vi "MenuDo.vi"(0 "GroupCol in":refnum<class "GroupCol.lvclass">, 1 "Column Array":refnum<vi>, 2 "Layout Ring Refnum":refnum<vi>, 3 "Clipboard":refnum<vi>, 5 "ItemTag":string, 7 "VariableManagerRef":refnum<vi>, 9 "Table CtlRef In":refnum<vi>, 11 "error in (no error)":errorcluster, 12 "Cell Position":T1, 13 "ModeCol Index":i32=2, 14 "Table History ref":refnum<vi>) -> (4 "GroupCol out":refnum<class "GroupCol.lvclass">, 6 "Col Array Ref out":refnum<vi>, 8 "Update HWI?":bool, 10 "Table CtlRef Out":refnum<vi>, 15 "error out":errorcluster)   [LabVIEW 2013, in "GroupCol.lvclass"]
doc: "Perform selected shortcut (right-click) menu actions for Group column.\nThis VI is read-only w.r.t column data."
uses:
  GroupCol.lvclass
  <vilib>/Utility/miscctls.llb/LVRowAndColumnTypeDef.ctl
  TypeDefs/TableHistory.ctl
  TypeDefs/TableArray.ctl
  VariableManagerCodes/VariableManager/VariableManager.lvclass
  DigitalCol/DigitalCol.lvclass
  Globals/StdRowHeightGlobal.vi
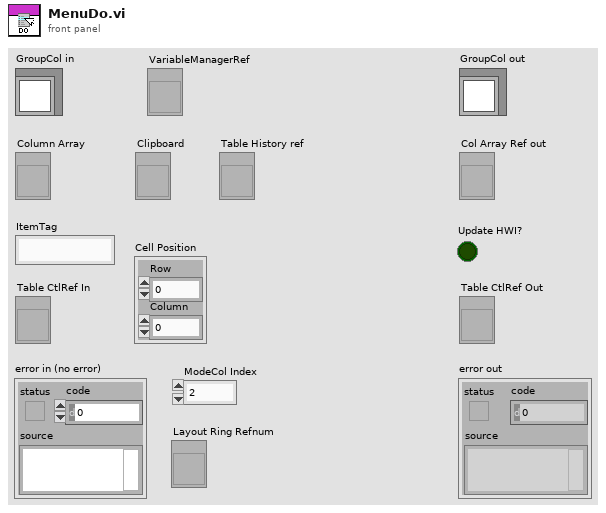
[diagram p1: front panel]
types:
  T1 = typedef "LVRowAndColumnTypeDef.ctl" = cluster{"Row":i32, "Column":i32}
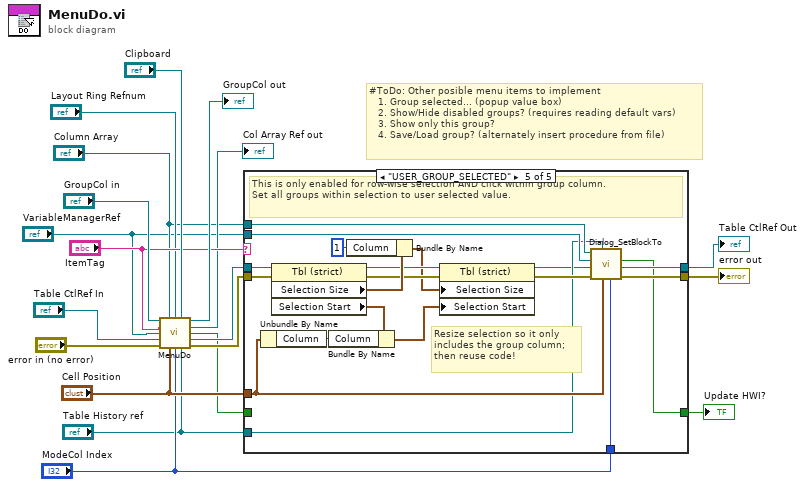
[diagram p0: block diagram]
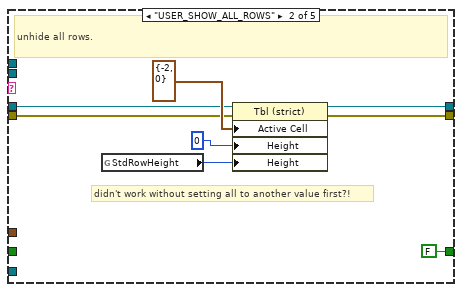
[diagram p3: hidden frame]
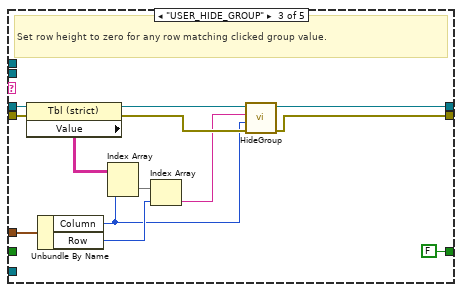
[diagram p4: hidden frame]
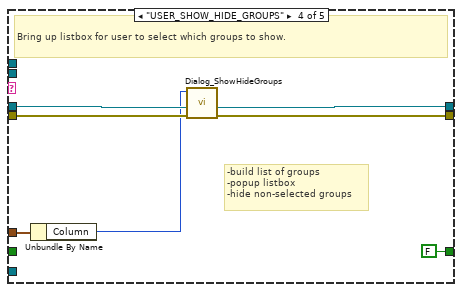
[diagram p5: hidden frame]
diagram:
  # "#ToDo: Other posible menu items to implement\n   1. Group selected... (popup value box)\n   2. Show/Hide disabled groups? (requires reading default vars)\n   3. Show only this group?\n   4. Save/Load group? (alternately insert procedure from file)"
  n1 = call-parent "MenuDo.vi"("DigitalCol in"="GroupCol in", "Column Array"="Column Array", "Layout Ring Refnum"="Layout Ring Refnum", "Clipboard"="Clipboard", "ItemTag"="ItemTag", "VariableManagerRef"="VariableManagerRef", "Table CtlRef In"="Table CtlRef In", "error in (no error)"="error in (no error)", "Cell Position"="Cell Position", "ModeCol Index"="ModeCol Index", "Table History ref"="Table History ref") -> ("DigitalCol out"=→"GroupCol out":refnum<class "GroupCol.lvclass">, "Col Array Ref out"=→"Col Array Ref out":refnum<vi>, "Update HWI?"=w2:bool, "Table CtlRef Out"=w9:refnum<vi>, "error out"=w10:errorcluster)
  n2 = case shown="\"USER_GROUP_SELECTED\"" "ItemTag" {
    tunnel: w9 -> [w22 w27 w42 w50 w69]
    tunnel: w10 -> [w21 w26 w39 w49 w68]
    tunnel: [w21 w30 w32 w48 w58] -> w19
    tunnel: [w22 w29 w43 w47 w52] -> w18
    tunnel: "Cell Position" -> [_ _ w36 w46 w57]
    tunnel: "ModeCol Index" -> [_ _ _ _ w56]
    tunnel: "Column Array" -> [_ _ _ _ w55]
    tunnel: "VariableManagerRef" -> [_ _ _ _ w54]
    tunnel: "Table History ref" -> [_ _ _ _ w53]
    tunnel: w2 -> [w20 _ _ _ _]
    tunnel: [w20 FALSE ("Update HWI?") FALSE ("Update HWI?") FALSE ("Update HWI?") w51] -> w1
    frame Default {
    }
    frame "USER_SHOW_ALL_ROWS" {
      # "didn't work without setting all to another value first?!"
      # "unhide all rows."
      n3 = global read "StdRowHeightGlobal.vi" "StdRowHeight"() -> (w25:u32)
      n4 = property class="Tbl (strict)"(reference=w27, error in=w26, "Active Cell"=T1 {"Row"=-2, "Column"=0} ("Active Cell:Active Cell"), "Height"=u32 0 ("Active Cell:Cell Size:Height"), "Height"=w25) -> (reference out=w29:refnum<vi>, error out=w30:errorcluster)
    }
    frame "USER_HIDE_GROUP" {
      # "Set row height to zero for any row matching clicked group value."
      n5 = property class="Tbl (strict)"(reference=w42, error in=w39) -> (reference out=w41:refnum<vi>, error out=w40:errorcluster, "Value"=w38:string[][])
      n6 = Unbundle By Name(w36) -> ("Column"=w33:i32, "Row"=w35:i32)
      n7 = Index Array(array=w38, index (col)=w33) -> (element=w37:string[])  [unwired: 1 in]
      n8 = Index Array(array=w37, index=w35) -> (element=w34:string)
      n9 = call "HideGroup.vi"("error in (no error)"=w40, "GroupCol Index"=w33, "String toHide"=w34, "Table CtlRef In"=w41) -> ("error out"=w32:errorcluster, "Table CtlRef Out"=w43:refnum<vi>)  [unwired: 6 in]
    }
    frame "USER_SHOW_HIDE_GROUPS" {
      # "-build list of groups\n-popup listbox\n-hide non-selected groups"
      # "Bring up listbox for user to select which groups to show."
      n10 = Unbundle By Name(w46) -> ("Column"=w45:i32)
      n11 = call "Dialog_ShowHideGroups.vi"("error in (no error)"=w49, "Table CtlRef In"=w50, "GroupCol Index"=w45) -> ("error out"=w48:errorcluster, "Table CtlRef Out"=w47:refnum<vi>)  [unwired: 7 in]
    }
    frame "USER_GROUP_SELECTED" {
      # "Resize selection so it only\nincludes the group column;\nthen reuse code!"
      # "This is only enabled for row-wise selection AND click within group column.\nSet all groups within selection to user selected value."
      n12 = Unbundle By Name(w57) -> ("Column"=w66:i32)
      n13 = property class="Tbl (strict)"(reference=w69, error in=w68) -> (reference out=w63:refnum<vi>, error out=w62:errorcluster, "Selection Size"=w65:T1, "Selection Start"=w67:T1)
      n14 = Bundle By Name(cluster=w67, "Column"=w66) -> (w60:T1)
      n15 = Bundle By Name(cluster=w65, "Column"=1 ("Row")) -> (w61:T1)
      n16 = property class="Tbl (strict)"(reference=w63, error in=w62, "Selection Size"=w61, "Selection Start"=w60) -> (reference out=w52:refnum<vi>, error out=w59:errorcluster)
      n17 = call "Dialog_SetBlockTo.vi"("ModeCol Index"=w56, "Cell Position"=w57, "Table History ref"=w53, "error in (no error)"=w59, "Table CtlRef In"=w52, "VariableManagerRef"=w54, "Col Array Ref in"=w55) -> ("error out"=w58:errorcluster, "OK"=w51:bool)  [unwired: 3 in]
    }
  }
  "error out" <- w19
  "Table CtlRef Out" <- w18
  "Update HWI?" <- w1
